vi "ClipPaning.vi"(3 "Error In":errorcluster, 5 "location":i32(ring) items=["left"=2250, "right"=-3500, "lock screw"=1345, "lock_nut"=1167, "push"=-2805, "middle"=0]) -> (10 "Error Out":errorcluster)   [LabVIEW 2019]
uses:
  <vilib>/Platform/TimedLoop/XDataNode/timing_clust.ctl
  <vilib>/Platform/TimedLoop/XDataNode/nitl_modes.ctl
  <vilib>/Platform/TimedLoop/XDataNode/wakeup.ctl
  WSCbot_V3_Toolkit.lvlibp/WSCBOTV3_Toolkit/IO/LowLevel/IO_Chanel_DIO.ctl
  WSCbot_V3_Toolkit.lvlibp/WSCBOTV3_Toolkit/IO/LowLevel/PulseCounter.ctl
  <vilib>/platform/TimedLoop/XDataNode/XDataNode.xnode
  WSCbot_V3_Toolkit.lvlibp
  <vilib>/Platform/TimedLoop/XDataNode/XDNodeRunTimeDep.lvlib
panel:
  in  "Stop Button":bool
  out "F710 button info.RB":bool
  out "Stop Output":bool
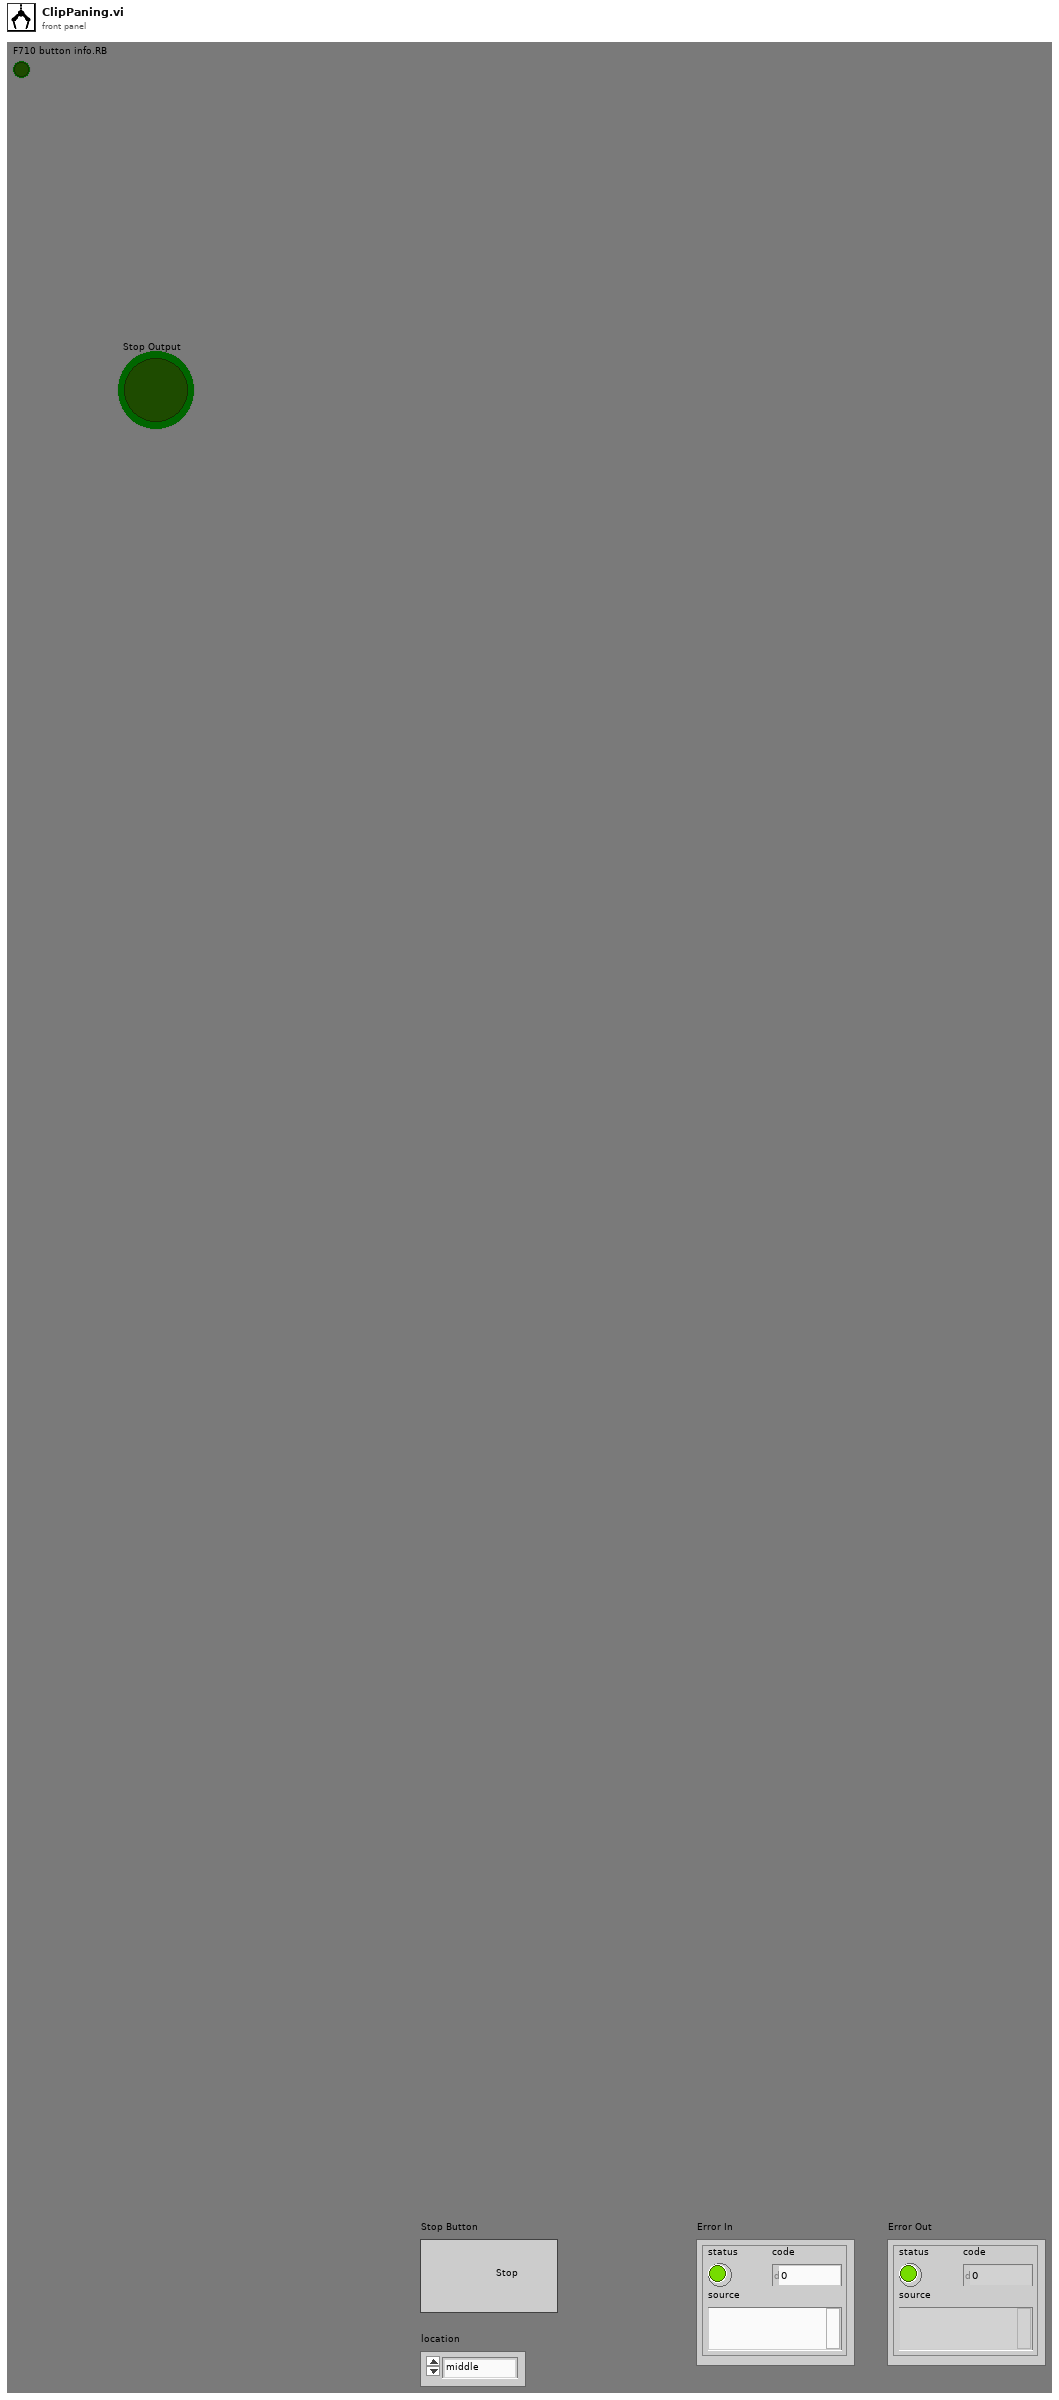
[diagram p1: front panel]
types:
  T1 = typedef "XDNodeRunTimeDep.lvlib/timing_clust.ctl" = cluster{"Expected End [f-1]":u64, "Actual End [f-1]":u64, "Finished Late? [f-1]":bool, "Expected End [i-1]":u64, "Actual End [i-1]":u64, "Finished Late? [i-1]":bool, "Expected Start [i]":u64, "Actual Start [i]":u64, "Expected Start [f]":u64, "Actual Start [f]":u64, "Source Name":string, "Structure Name":string, "Period":i64, "Deadline":i64, "Offset":i64, "Start":i64, "Priority":i32, "Timeout":i32, "Mode":T2, "Wakeup Reason":T3, "Error":errorcluster, "Source Type":string, "Secondary Source Type":string, "Global End Time":u64, "Global Start Time":u64, "Frame Duration":u64, "Iteration Duration":u64, "Assigned CPU":i32, "I/O Scan Engine Mode":u32}
  T2 = typedef "XDNodeRunTimeDep.lvlib/nitl_modes.ctl" = enum32{"No Change", "Process missed periods, maintain original phase", "Discard missed periods, maintain original phase", "Process missed periods, ignore original phase", "Discard missed periods, ignore original phase"}
  T3 = typedef "XDNodeRunTimeDep.lvlib/wakeup.ctl" = enum32{"Normal", "Aborted", "Asynchronous wakeup", "Timing source error", "Timed loop error", "Timeout"}
  T4 = typedef "WSCbot_V3_Toolkit.lvlibp/PulseCounter.ctl" = enum16{"CH1", "CH2", "CH3", "CH4", "CH5"}
  T5 = typedef "WSCbot_V3_Toolkit.lvlibp/IO_Chanel_DIO.ctl" = enum16{"A/DIO9", "A/DIO10", "C/DIO0", "C/DIO1", "C/DIO2", "C/DIO3", "C/DIO4", "C/DIO5", "C/DIO6"}
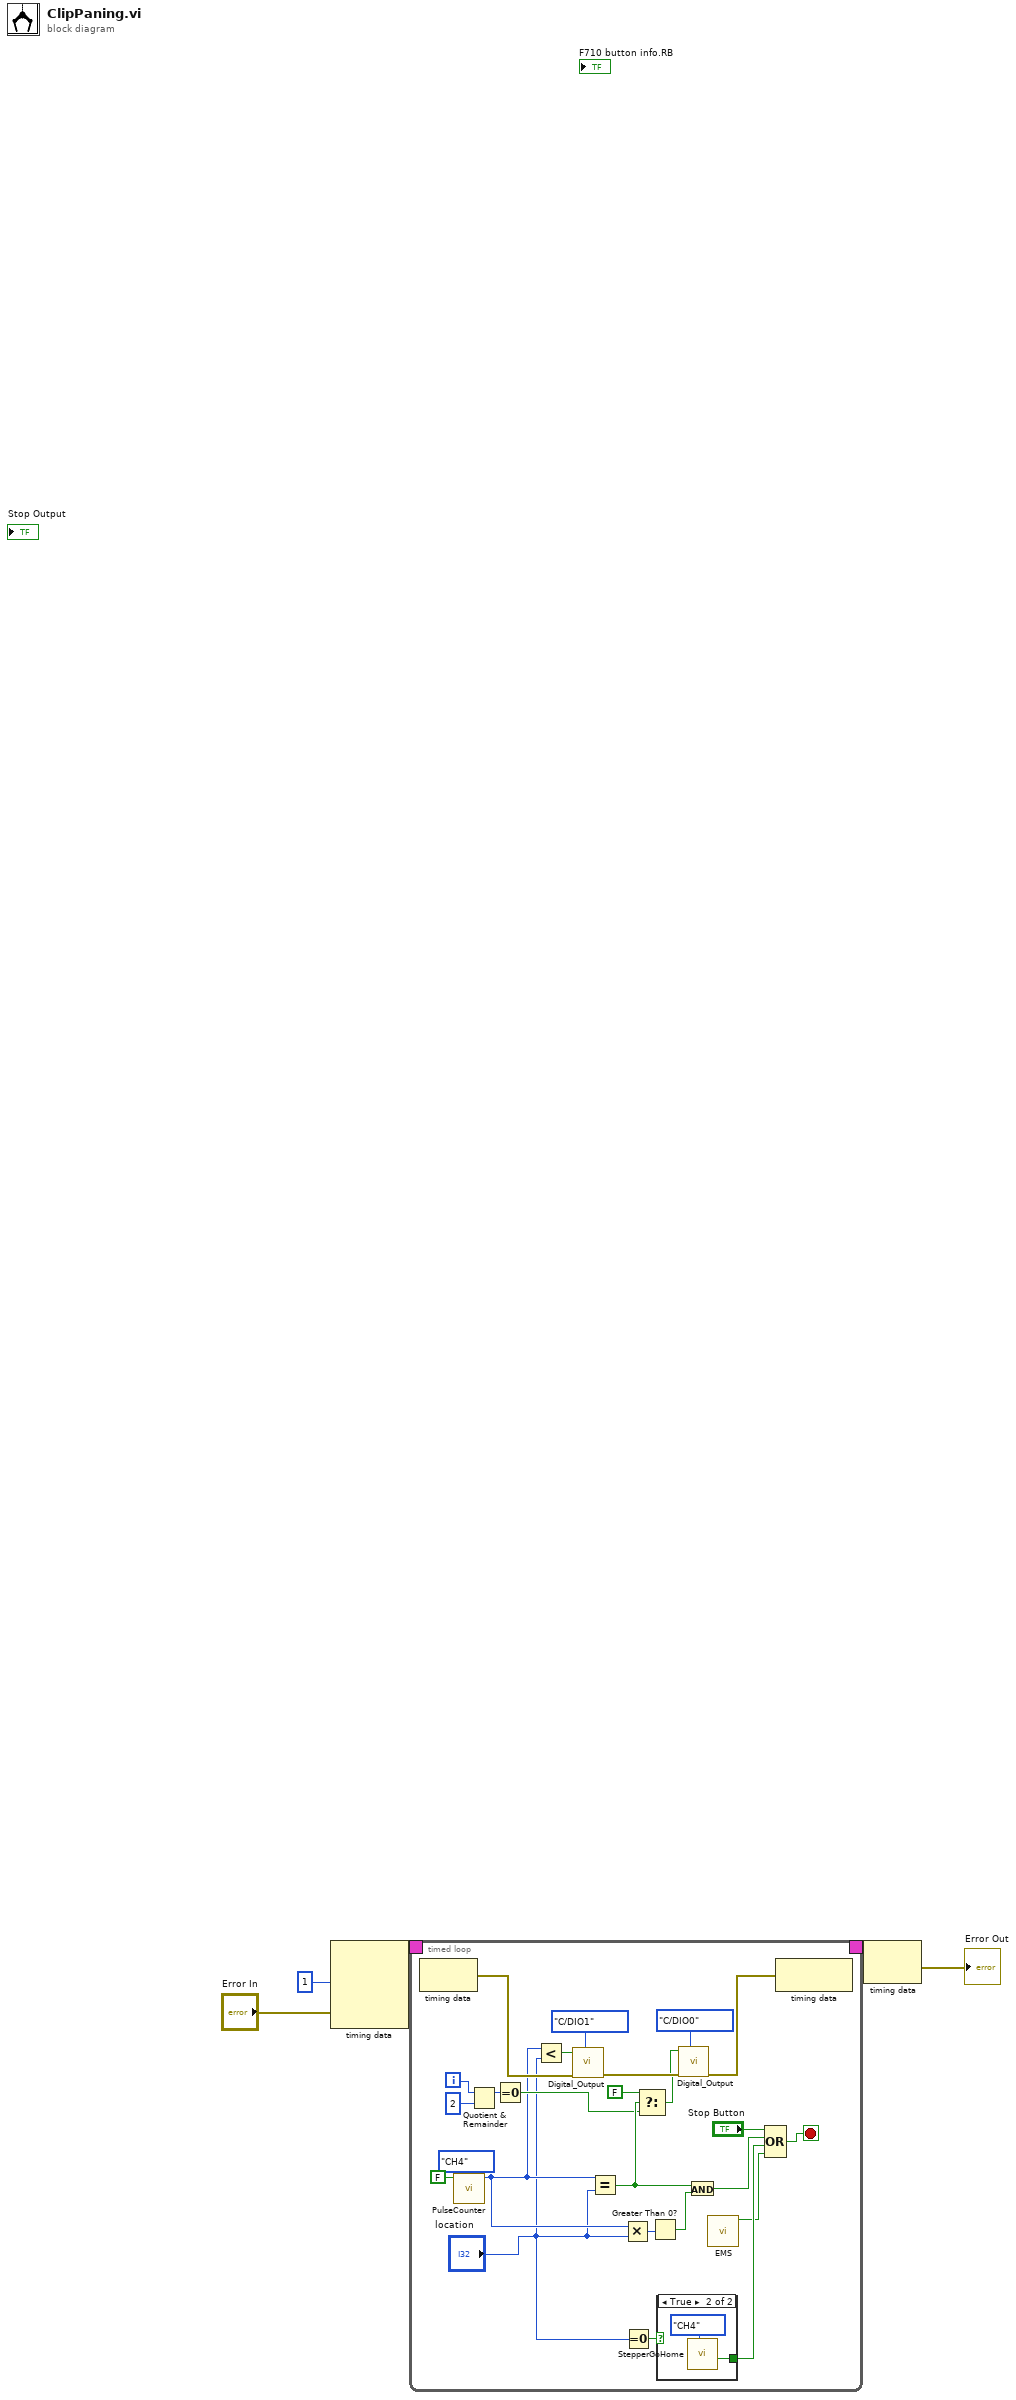
[diagram p0: block diagram]
diagram:
  n1 = node-c288(i64 1 ("Period"), "Error In") -> (w5:T1)  [unwired: 2 in]
  n2 = timed-loop {
    timing: w5 -> [_]
    timing-out: [_] -> w4
    i -> [w25]
    stop <- w21 stop-if-true
    n3 = node-c288() -> (w24:errorcluster)  [unwired: 1 in]
    n4 = call "PulseCounter.vi"("PulseCounterChanel"=PulseCounter."CH4", "Reset"=FALSE) -> ("PulseCount"=w10:i32)  [unwired: 8 in, 1 out]
    n5 = Quotient & Remainder(x=w25, y=2) -> (x-y*floor(x/y)=w26:i32)  [unwired: 1 out]
    n6 = Equal To 0?(x=w26) -> (x = 0?=w13:bool)
    n7 = Less?(x=w10, y="location") -> (x < y?=w19:bool)
    n8 = call "Digital_Output.vi"("IO_Chanel"=IO_Chanel_DIO."C/DIO1", "error in"=w24, "False/True"=w19) -> ("error out"=w29:errorcluster)  [unwired: 8 in]
    n9 = Equal?(x=w10, y="location") -> (x = y?=w14:bool)
    n10 = Multiply(x=w10, y="location") -> (x*y=w17:i32)
    n11 = Equal To 0?(x="location") -> (x = 0?=w18:bool)
    n12 = Select(t=FALSE, s=w14, f=w13) -> (s? t:f=w11:bool)
    n13 = Greater Than 0?(x=w17) -> (x > 0?=w16:bool)
    n14 = case shown="True" w18 {
      selector: w18 -> [w31 _]
      tunnel: [w31 w32] -> w15
      frame False {
      }
      frame True {
        n15 = call "StepperGoHome.vi"("PulseCounterChanel"=PulseCounter."CH4") -> ("stop output"=w32:bool)  [unwired: 8 in, 2 out]
      }
    }
    n16 = call "Digital_Output.vi"("IO_Chanel"=IO_Chanel_DIO."C/DIO0", "error in"=w29, "False/True"=w11) -> ("error out"=w23:errorcluster)  [unwired: 8 in]
    n17 = And(x=w14, y=w16) -> (x .and. y?=w8:bool)
    n18 = call "EMS.vi"() -> ("EMS"=w7:bool)  [unwired: 10 in, 1 out]
    n19 = Compound Arithmetic op=OR("Stop Button", w8, w15, w7) -> (w21:bool)
    n20 = node-c288(w23) -> ()  [unwired: 1 out]
  }
  n21 = node-c288(w4) -> (→"Error Out":errorcluster)
